vi "SD Write Name Cache.vi"(8 "Field Value In":T1, 10 "Name":string, 11 "Table Prefix":string) -> (0 "Field Value Out":T1)   [LabVIEW 2017]
uses:
  <vilib>/Rock Robotics/Network Tables/Field Data.ctl
  <vilib>/Rock Robotics/Network Tables/Field Type.ctl
  <vilib>/Rock Robotics/Network Tables/Sequence.ctl
  <vilib>/Rock Robotics/Network Tables/Make Table Operation.ctl
  <vilib>/Rock Robotics/Network Tables/Manage Dirty Field ID List.vi
  <vilib>/Rock Robotics/Network Tables/NT Globals.vi
  <vilib>/Rock Robotics/Network Tables/Update Other Clients.vi
  <vilib>/Rock Robotics/Network Tables/Build Entry Assign Buffer.vi
  <vilib>/Rock Robotics/Network Tables/Field Data Manager.vi
  <vilib>/Rock Robotics/Network Tables/Usage Statistics.vi
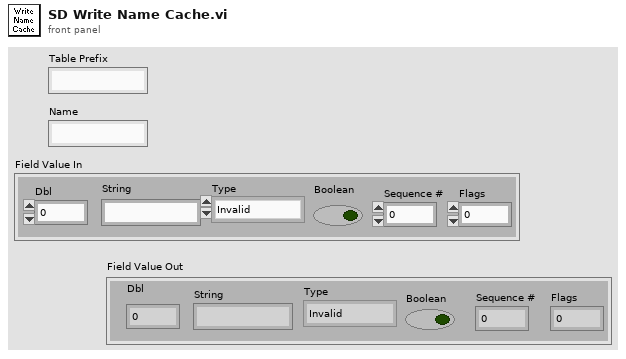
[diagram p1: front panel]
types:
  T1 = typedef "Field Data.ctl" = cluster{"Dbl":dbl, "String":string, "Type":T2, "Boolean":bool, "Sequence #":T3, "Flags":u8}
  T2 = typedef "Field Type.ctl" = enum8{"Invalid", "Bool", "Numeric", "String", "Raw", "Boolean Array", "Numeric Array", "String Array", "RPC"}
  T3 = typedef "Sequence.ctl" = u16
  T4 = typedef "Make Table Operation.ctl" = enum16{"Get or Add Field", "Get Field or Add Temp", "Replace Temp ID", "Get Field ID - No Add", "Get Table Field IDs", "Get Field ID Info", "Move Field to Temp", "Validate", "Remove Field", "Remove All"}
  T5 = typedef "Field ID.ctl" = i32
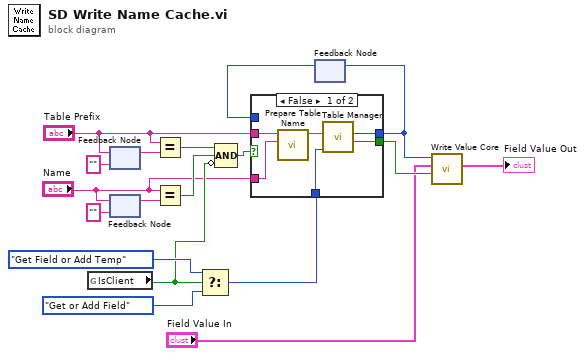
[diagram p0: block diagram]
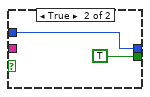
[diagram p2: hidden frame]
diagram:
  n1 = global read "NT Globals.vi" "IsClient"() -> (w8:bool)
  n2 = feedback-in #1("Table Prefix") -> ()
  n3 = feedback #1("" ("Name")) -> (w13:string)
  n4 = feedback #2("" ("Name")) -> (w3:string)
  n5 = feedback-in #2("Name") -> ()
  n6 = Equal?(x="Table Prefix", y=w13) -> (x = y?=w9:bool)
  n7 = Equal?(x="Name", y=w3) -> (x = y?=w2:bool)
  n8 = Select(t=Make_Table_Operation."Get Field or Add Temp" ("Operation"), s=w8, f=Make_Table_Operation."Get or Add Field" ("Operation")) -> (s? t:f=w18:T4)
  n9 = Compound Arithmetic op=AND(w9, w2, invert w8) -> (w7:bool)
  n10 = feedback #3() -> (w10:T5)  [unwired: 1 in]
  n11 = case shown="False" w7 {
    tunnel: w18 -> [w24 _]
    tunnel: [w23 TRUE ("Success")] -> w15
    tunnel: [w22 w26] -> w11
    tunnel: "Table Prefix" -> [w20 _]
    tunnel: w10 -> [_ w26]
    tunnel: "Name" -> [w19 _]
    frame False {
      n12 = call <vilib>:"Prepare Table Name.vi"("Name"=w19, "Table Prefix"=w20) -> ("Prefixed Name"=w21:string)  [unwired: 9 in]
      n13 = call <vilib>:"Table Manager.vi"("Operation"=w24, "Entry Name"=w21) -> ("Success"=w23:bool, "Entry ID"=w22:T5)  [unwired: 6 in, 2 out]
    }
    frame True {
    }
  }
  n14 = feedback-in #3(w11) -> ()
  n15 = call <vilib>:"Write Value Core.vi"("Existing"=w15, "Field Value"="Field Value In", "Field ID"=w11) -> ("Field Value Out"=→"Field Value Out":T1)  [unwired: 8 in]
